vi "Import Configuration File.vi"(8 "error in":errorcluster, 10 "parameters configuration file path":path caption="path to parameters xml", 11 "Ballard MIL-STD 1553 custom device in":T1 format="%.0x") -> (0 "error out":errorcluster, 3 "Ballard MIL-STD 1553 custom device out":T1 format="%.0x")   [LabVIEW 2020, in "Ballard MIL-STD-1553 Scripting.lvlib"]
doc: "For the specified <b>Ballard MIL-STD-1553 custom device in</b>, imports the parameters configuration file located at the input <b>parameters configuration file path</b>. For successful deployment and operation, the parameters configuration must be consistent with the hardware configuration."
uses:
  Ballard MIL-STD-1553 Scripting.lvlib
  <vilib>/NI VeriStand/Custom Device API/Custom Device Item Ref.ctl
  Import/MIL-STD 1553 Import.lvlib
  <vilib>/NI VeriStand/Custom Device API/Custom Device API.lvlib
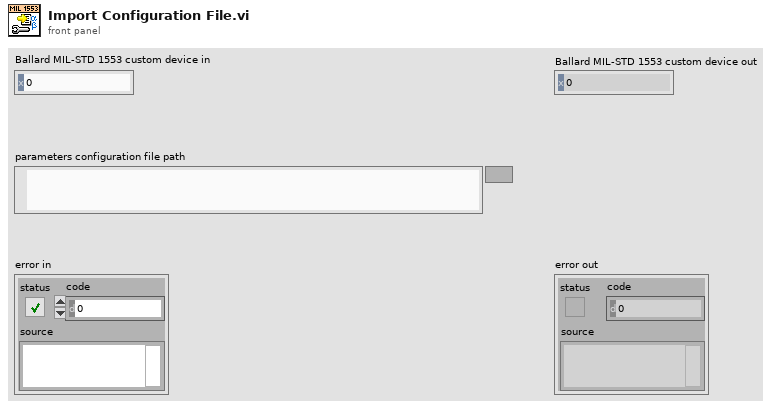
[diagram p1: front panel]
types:
  T1 = typedef "Custom Device API.lvlib/Custom Device Item Ref.ctl" = u64
  T2 = typedef "1553 Channel.ctl" = cluster{"HW channel":u16, "terminals":T3[], "messages":T5[], "acyclic frame names":string[]}
  T3 = typedef "Terminal Name and Address.ctl" = cluster{"name":string, "terminal address":T4}
  T4 = typedef "Address.ctl" = u16
  T5 = typedef "Message Definition.ctl" = cluster{"name":string, "message type":T6, "endpoint Rx":T7, "endpoint Tx":T7, "mode code":u16, "number of words":u16, "parameters":cluster{"name":string, "default value":dbl, "unit":string, "parameter definition":T8}[], "create timestamp channel":bool}
  T6 = typedef "Message Type.ctl" = string
  T7 = typedef "Terminal Endpoint.ctl" = cluster{"terminal address":T4, "subaddress":T4}
  T8 = typedef "Parameter Definition.ctl" = cluster{"start index":i32, "size (bits)":i32, "encoding":enum16{"BNR", "BCD", "Discrete"}, "signed":bool, "multiplier":dbl, "offset":dbl}
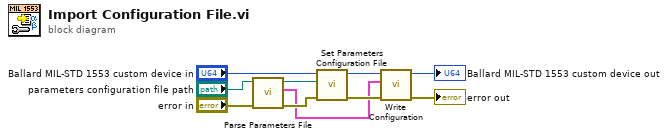
[diagram p0: block diagram]
diagram:
  n1 = call "Parse Parameters File.vi"("error in"="error in", "path to XML document"="parameters configuration file path") -> ("error out"=w7:errorcluster, "1553 channels"=w1:T2[], "path to XML document out"=w8:path)  [unwired: 7 in]
  n2 = call "Set Parameters Configuration File.vi"("error in"=w7, "parameters configuration file path"=w8, "Ballard MIL-STD 1553 custom device in"="Ballard MIL-STD 1553 custom device in") -> ("error out"=w9:errorcluster, "Ballard MIL-STD 1553 custom device out"=w10:T1)  [unwired: 7 in]
  n3 = call "Write Configuration.vi"("error in"=w9, "1553 channels"=w1, "Ballard MIL-STD 1553 custom device in"=w10) -> ("error out"=→"error out":errorcluster, "Ballard MIL-STD 1553 custom device out"=→"Ballard MIL-STD 1553 custom device out":T1)  [unwired: 7 in]
